vi "REQ Making Connection.vi"(8 "error in":errorcluster, 9 "Second Connection":cluster{"channel 3":string, "channel 4":string}={"channel 3"="r1", "channel 4"="c1"}, 10 "First Connection":cluster{"channel 1":string, "channel 2":string}={"channel 1"="r0", "channel 2"="c0"}) -> (0 "error out":errorcluster)   [LabVIEW 2016, in "S-Matrix.lvlib"]
doc: "_____\nCreated using DQMH Event Scripter 6.1.0.128."
uses:
  S-Matrix.lvlib
  REQ Making Connection Argument--cluster.ctl
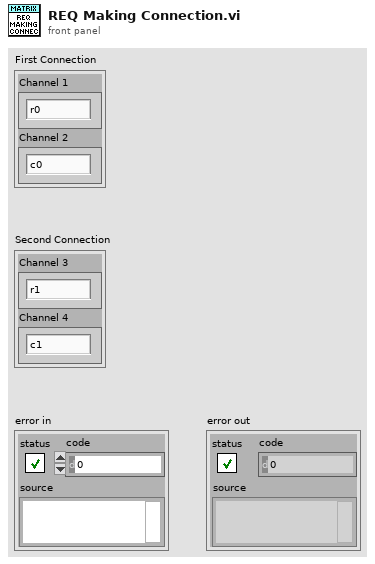
[diagram p1: front panel]
types:
  T1 = typedef "S-Matrix.lvlib/REQ Making Connection Argument--cluster.ctl" = cluster{"First Connection":cluster{"channel 1":string, "channel 2":string}, "Second Connection":cluster{"channel 3":string, "channel 4":string}}
  T2 = typedef "S-Matrix.lvlib/Request Events--cluster.ctl" = cluster{"Stop Module":refnum<user-event>, "Show Panel":refnum<user-event>, "Hide Panel":refnum<user-event>, "Get Module Execution Status":refnum<user-event>, "Show Diagram":refnum<user-event>, "REQ Initialize Hardware":refnum<user-event>, "REQ Single Relay":refnum<user-event>, "REQ Close Ref":refnum<user-event>, "REQ Making Connection":refnum<user-event>, "REQ Disconnect Channel":refnum<user-event>}
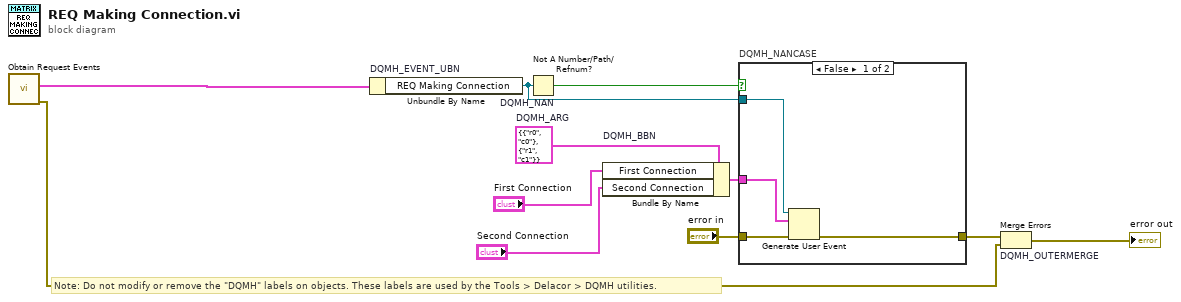
[diagram p0: block diagram]
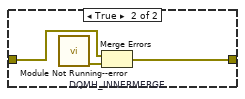
[diagram p2: hidden frame]
diagram:
  w5 = T1 {"First Connection"={"channel 1"="r0", "channel 2"="c0"}, "Second Connection"={"channel 3"="r1", "channel 4"="c1"}}  # DQMH_ARG
  # "Note: Do not modify or remove the \"DQMH\" labels on objects. These labels are used by the Tools > Delacor > DQMH utilities."
  n1 = call "Obtain Request Events.vi"() -> ("error out"=w2:errorcluster, "S-Matrix Request Events"=w1:T2)  [unwired: 10 in]
  n2 = Unbundle By Name "DQMH_EVENT_UBN"(w1) -> ("REQ Making Connection"=w7:refnum<user-event>)
  n3 = Not A Number/Path/Refnum? "DQMH_NAN"(number/path/refnum=w7) -> (NaN/Path/Refnum?=w8:bool)
  n4 = Bundle By Name "DQMH_BBN"(cluster=w5, "First Connection"="First Connection", "Second Connection"="Second Connection") -> (w9:T1)
  n5 = case "DQMH_NANCASE" shown="False" w8 {
    tunnel: "error in" -> [w15 w18]
    tunnel: [w14 w17] -> w6
    tunnel: w7 -> [w13 _]
    tunnel: w9 -> [w12 _]
    frame False {
      n6 = Generate User Event(user event=w13, event data cluster=w12, error in=w15) -> (error out=w14:errorcluster)  [unwired: 1 in, 1 out]
    }
    frame True {
      n7 = call "Module Not Running--error.vi"() -> ("error out"=w16:errorcluster)  [unwired: 11 in]
      n8 = Merge Errors "DQMH_INNERMERGE"(w18, w16) -> (w17:errorcluster)
    }
  }
  n9 = Merge Errors "DQMH_OUTERMERGE"(w6, w2) -> (→"error out":errorcluster)
